vi "PART_II.vi"() -> ()   [LabVIEW 2019]
uses:
  <vilib>/Utility/file.llb/Read Delimited Spreadsheet (DBL).vi
panel:
  in  "n":i32
  out "Low Event Index":i32[](array[numeric])
  out "High Event Index":i32[](array[numeric])
  out "Low Event Data":dbl[](array[numeric])
  out "High Event Data":dbl[](array[numeric])
  in  "stop":bool
  in  "threshold":dbl
  out "subarray":dbl[](array[numeric])
  in  "file path (dialog if empty)":path
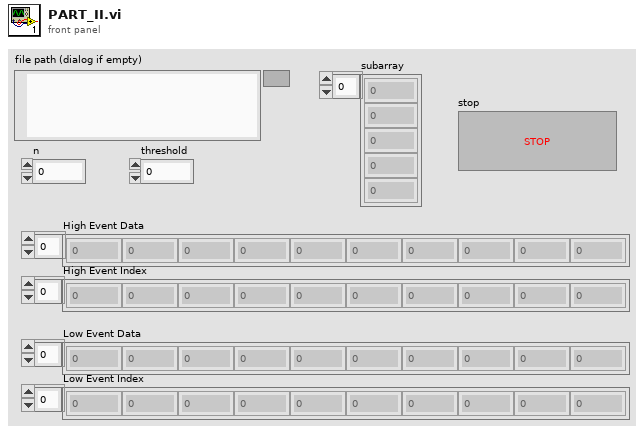
[diagram p1: front panel]
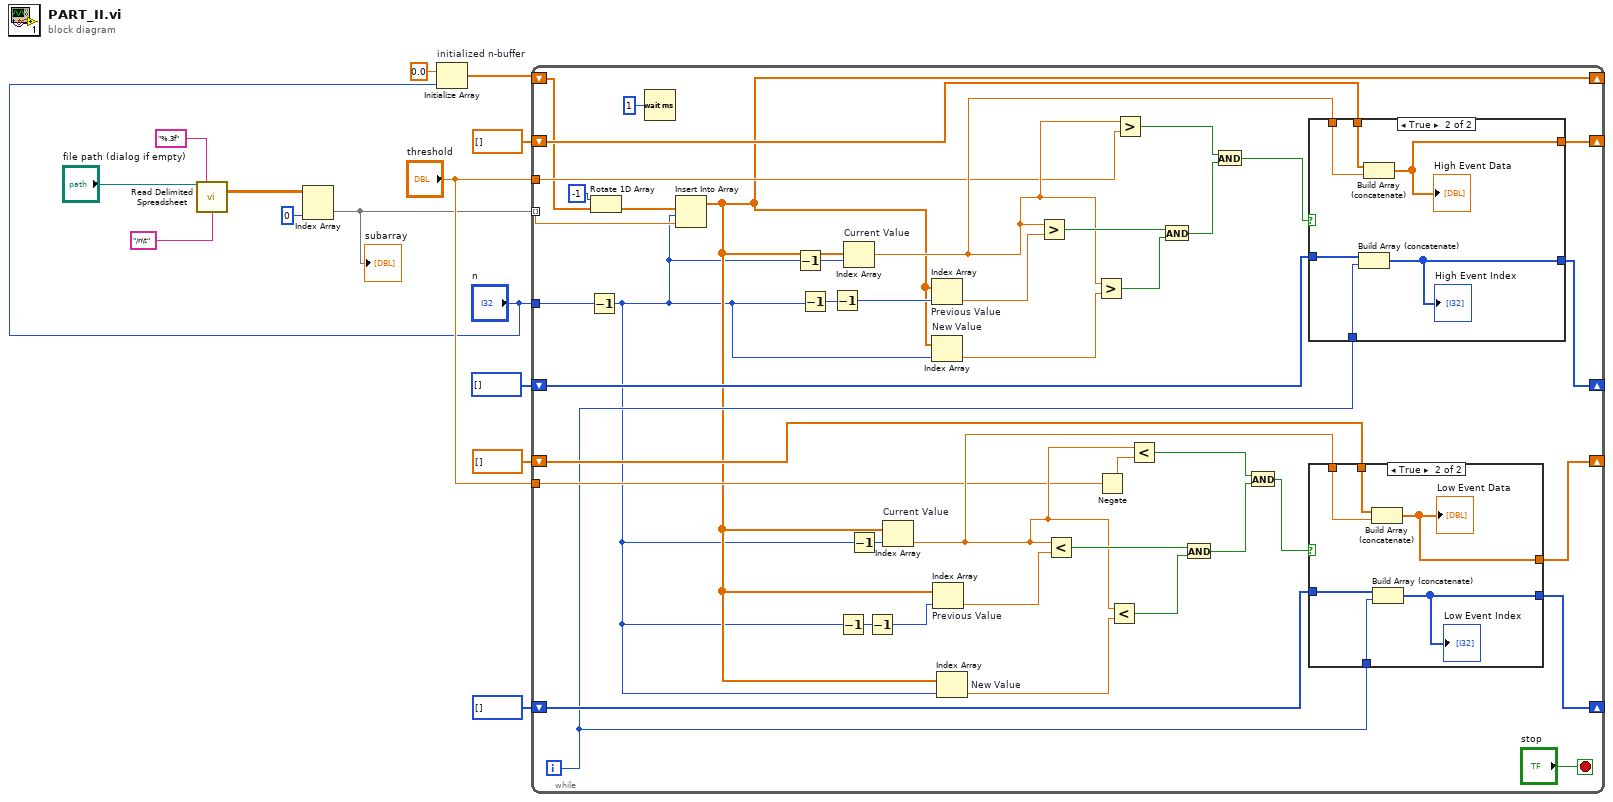
[diagram p0: block diagram]
diagram:
  n1 = call-poly <vilib>:"Read Delimited Spreadsheet.vi"("file path (dialog if empty)"="file path (dialog if empty)", "format (%.3f)"="%.3f", "delimiter (\\t)"="/n\t" ("delimiter (\\t)")) -> ("all rows"=w11:dbl[][])  [unwired: 7 in, 5 out]
  n2 = Index Array(array=w11, index (col)=0 ("disabled index (col)")) -> (element=w4:dbl[])  [unwired: 1 in]
  "subarray" <- w4
  n3 = Initialize Array "initialized n-buffer"(0.0 ("element"), "n") -> (w1:dbl[])
  n4 = while {
    tunnel: w4 -> [w19] mode=indexing
    shift-right: [w46] -> _
    shift-left: dbl[] [] -> [w45]
    shift-right: [w44] -> _
    shift-left: i32[] [] -> [w43]
    shift-right: [w33] -> _
    shift-left: dbl[] [] -> [w32]
    shift-right: [w31] -> _
    shift-left: i32[] [] -> [w30]
    tunnel: "threshold" -> [w28]
    tunnel: "threshold" -> [w27]
    shift-right: [w18] -> _
    shift-left: w1 -> [w25]
    tunnel: "n" -> [w22]
    i -> [w26]
    stop <- "stop" stop-if-true
    n5 = Decrement(x=w22) -> (x-1=w15:i32)
    n6 = Rotate 1D Array(1:w25, 2:-1 ("n")) -> (0:w23:dbl[])
    n7 = Wait (ms)(milliseconds to wait=u32 1) -> ()  [unwired: 1 out]
    n8 = Insert Into Array(array=w23, index=w15, new element=w19) -> (w18:dbl[])
    n9 = Decrement(x=w15) -> (x-1=w20:i32)
    n10 = Decrement(x=w15) -> (x-1=w21:i32)
    n11 = Decrement(x=w21) -> (x-1=w51:i32)
    n12 = Decrement(x=w15) -> (x-1=w42:i32)
    n13 = Index Array "Current Value"(array=w18, index=w20) -> (element=w47:dbl)
    n14 = Decrement(x=w15) -> (x-1=w16:i32)
    n15 = Decrement(x=w42) -> (x-1=w17:i32)
    n16 = Index Array "Current Value"(array=w18, index=w16) -> (element=w34:dbl)
    n17 = Index Array "Previous Value"(array=w18, index=w51) -> (element=w57:dbl)
    n18 = Index Array "New Value"(array=w18, index=w15) -> (element=w56:dbl)
    n19 = Index Array "Previous Value"(array=w18, index=w17) -> (element=w41:dbl)
    n20 = Index Array "New Value"(array=w18, index=w15) -> (element=w40:dbl)
    n21 = Greater?(x=w47, y=w57) -> (0:w55:bool)
    n22 = Less?(x=w34, y=w41) -> (x < y?=w39:bool)
    n23 = Greater?(x=w47, y=w56) -> (0:w54:bool)
    n24 = Negate(x=w27) -> (-x=w29:dbl)
    n25 = Less?(x=w34, y=w40) -> (x < y?=w38:bool)
    n26 = Greater?(x=w47, y=w28) -> (0:w53:bool)
    n27 = Less?(x=w34, y=w29) -> (x < y?=w37:bool)
    n28 = And(x=w55, y=w54) -> (x .and. y?=w52:bool)
    n29 = And(x=w39, y=w38) -> (x .and. y?=w36:bool)
    n30 = And(x=w53, y=w52) -> (x .and. y?=w49:bool)
    n31 = And(x=w37, y=w36) -> (x .and. y?=w35:bool)
    n32 = case shown="True" w49 {
      tunnel: w47 -> [_ w73]
      tunnel: [w67 w72] -> w46
      tunnel: w45 -> [w67 w71]
      tunnel: w26 -> [_ w70]
      tunnel: [w66 w69] -> w44
      tunnel: w43 -> [w66 w68]
      frame False {
      }
      frame True {
        n33 = Build Array (concatenate)(w68, w70) -> (w69:i32[])
        "High Event Index" <- w69
        n34 = Build Array (concatenate)(w71, w73) -> (w72:dbl[])
        "High Event Data" <- w72
      }
    }
    n35 = case shown="True" w35 {
      tunnel: w34 -> [_ w65]
      tunnel: [w59 w64] -> w33
      tunnel: w32 -> [w59 w63]
      tunnel: [w58 w62] -> w31
      tunnel: w26 -> [_ w61]
      tunnel: w30 -> [w58 w60]
      frame False {
      }
      frame True {
        n36 = Build Array (concatenate)(w63, w65) -> (w64:dbl[])
        "Low Event Data" <- w64
        n37 = Build Array (concatenate)(w60, w61) -> (w62:i32[])
        "Low Event Index" <- w62
      }
    }
  }
